vi "DS402 Drive - Get Virtual Channel VS refs.vi"(8 "Fehler (Eingang, kein Fehler)":errorcluster, 9 "Section Name":string, 10 "Item Ref":T1 format="%.0x", 11 "I/O Variable Data in":T2[](array[typedef]) {"VS ref" format="%.0x"}) -> (0 "Fehler (Ausgang)":errorcluster, 2 "Channel Refs":T1[](array[typedef]) format="%.0x", 3 "I/O Variable Data out":T2[](array[typedef]) {"VS ref" format="%.0x"})   [LabVIEW 2016, in "Scan Engine Custom Device.lvlib"]
uses:
  Scan Engine Custom Device.lvlib
  <vilib>/NI Veristand/Custom Device API/Custom Device Item Ref.ctl
  Type Defs/DS402 Drive ECAT Slave IOV Cluster.ctl
  Type Defs/UDV Data Type.ctl
  Globals/Property Strings.vi
  <vilib>/NI Veristand/Custom Device API/Get Item Property (I32).vi
  <vilib>/NI Veristand/Custom Device API/Custom Device API.lvlib
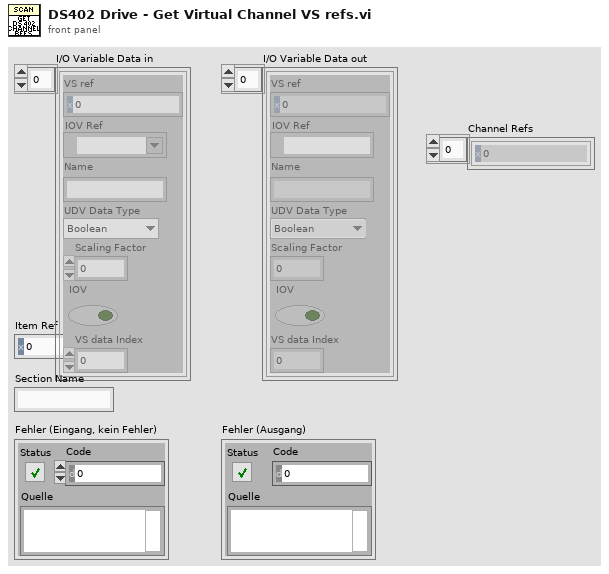
[diagram p1: front panel]
types:
  T1 = typedef "Custom Device API.lvlib/Custom Device Item Ref.ctl" = u64
  T2 = typedef "Scan Engine Custom Device.lvlib/DS402 Drive ECAT Slave IOV Cluster.ctl" = cluster{"VS ref":T1, "IOV Ref":refnum<k21>, "Name":string, "UDV Data Type":T3, "Scaling Factor":dbl, "IOV":bool, "VS data Index":i32}
  T3 = typedef "Scan Engine Custom Device.lvlib/UDV Data Type.ctl" = enum16{"Boolean", "Fixed Point", "Int8", "Int16", "Int32", "Int64", "U32 Bit Field", "UInt8", "UInt16", "UInt32", "UInt64", "Other"}
  T4 = typedef "Custom Device API.lvlib/Custom Device Item Info.ctl" = cluster{"Name":string, "Is Channel":bool, "GUID":string, "Is Waveform":bool}
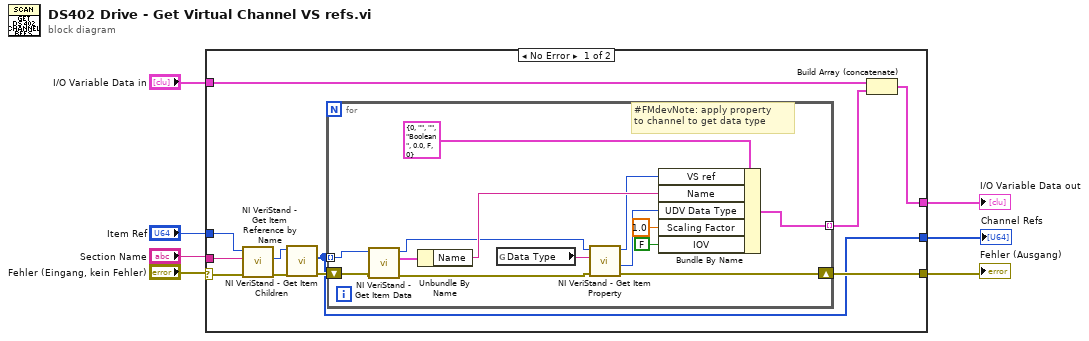
[diagram p0: block diagram]
diagram:
  n1 = case shown="No Error" "Fehler (Eingang, kein Fehler)" {
    selector: "Fehler (Eingang, kein Fehler)" -> [w13 w34]
    tunnel: "Item Ref" -> [w18 _]
    tunnel: [w9 w33] -> w6
    tunnel: [w17 w34] -> w5
    tunnel: "I/O Variable Data in" -> [w10 w33]
    tunnel: "Section Name" -> [w12 _]
    tunnel: [w11 _] -> w1
    frame No Error {
      n2 = call <vilib>:"NI VeriStand - Get Item Reference by Name.vi"("error in (no error)"=w13, "Item Name"=w12, "Parent Ref in"=w18) -> ("error out"=w15:errorcluster, "Item Ref"=w14:T1)  [unwired: 5 in, 2 out]
      n3 = call <vilib>:"NI VeriStand - Get Item Children.vi"("error in (no error)"=w15, "Item Ref in"=w14) -> ("error out"=w16:errorcluster, "Child Refs"=w11:T1[])  [unwired: 6 in, 2 out]
      n4 = for {
        tunnel: w11 -> [w31] mode=indexing
        shift-right: [w21] -> w17
        shift-left: w16 -> [w30]
        tunnel: [w29] -> w8 mode=indexing
        # "#FMdevNote: apply property \nto channel to get data type"
        n5 = call <vilib>:"NI VeriStand - Get Item Data.vi"("error in (no error)"=w30, "Item Ref in"=w31) -> ("error out"=w25:errorcluster, "Item Info"=w28:T4, "Item Ref out"=w24:T1)  [unwired: 6 in, 1 out]
        n6 = Unbundle By Name(w28) -> ("Name"=w27:string)
        n7 = global read "Property Strings.vi" "Data Type"() -> (w26:string)
        n8 = call-poly <vilib>:"NI VeriStand - Get Item Property.vi"("error in (no error)"=w25, "Property Name"=w26, "Item Ref in"=w24) -> ("error out"=w21:errorcluster, "Value"=w22:i32, "Item Ref out"=w23:T1)  [unwired: 5 in, 1 out]
        n9 = Bundle By Name(cluster=T2 {"VS ref"=0, "IOV Ref"="", "Name"="", "UDV Data Type"=enum."Boolean", "Scaling Factor"=0.0, "IOV"=FALSE, "VS data Index"=0} ("element"), "VS ref"=w23, "Name"=w27, "UDV Data Type"=w22, "Scaling Factor"=1.0, "IOV"=FALSE) -> (w29:T2)
      }
      n10 = Build Array (concatenate)(w10, w8) -> (w9:T2[])
    }
    frame Error {
    }
  }
  "I/O Variable Data out" <- w6
  "Fehler (Ausgang)" <- w5
  "Channel Refs" <- w1
